vi "1C Camera - find boat given marker locations.vi"(0 "Bow Marker Found":T1, 1 "Bow Marker Location":T3 {"North" format="%#_10f"; "East" format="%#_8f"}, 2 "Bow Marker Heading":T2 format="%05.1f", 3 "Stern Marker Found":T1, 4 "Stern Marker Location":T3 {"North" format="%#_10f"; "East" format="%#_8f"}, 5 "Stern Marker Heading":T2 format="%05.1f") -> (14 "Boat Location":T3 {"North" format="%#_10f"; "East" format="%#_8f"}, 15 "Heading":T2 format="%05.1f", 18 "Boat Found":T1)   [LabVIEW 2011]
doc: "Takes the information from two marker-finders, one for the bow and one for stern of the boat, and uses them to estimate the position of the center of the boat. \nAssumes that the center of the boat is either:\na. halfway in between the markers if both are found\nb. half of a boat length extrapolated in the appropriate direction from the marker that was found, if only one marker was found.\nIf neither marker was found, the Boat Found output will be False and you'll have to look elsewhere for your boat location information, sorry."
uses:
  2-Think/2 Typedefs/UTM Location.ctl
  2-Think/2 Typedefs/heading.ctl
  2-Think/2 Typedefs/indicator LED.ctl
  2-Think/2 Typedefs/Velocity.ctl
panel:
  in  "Distance Bow to Stern (m)":dbl=1.0
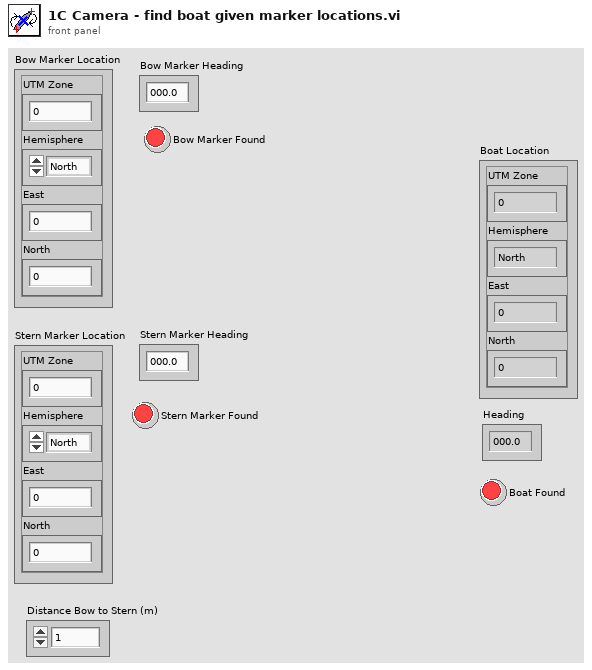
[diagram p1: front panel]
types:
  T1 = typedef "indicator LED.ctl" = bool
  T2 = typedef "heading.ctl" = dbl
  T3 = typedef "UTM Location.ctl" = cluster{"UTM Zone":dbl, "Hemisphere":enum16{"North", "South"}, "East":dbl, "North":dbl}
  T4 = typedef "Velocity.ctl" = cluster{"East":dbl, "North":dbl}
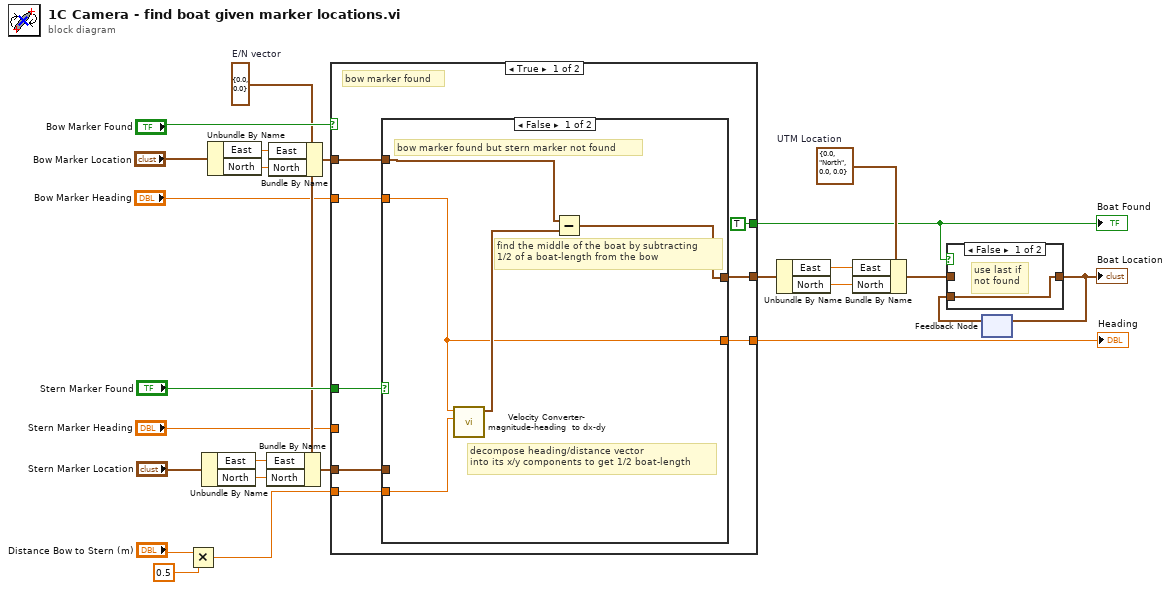
[diagram p0: block diagram]
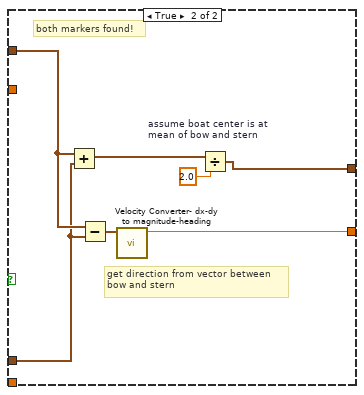
[diagram p3: hidden frame]
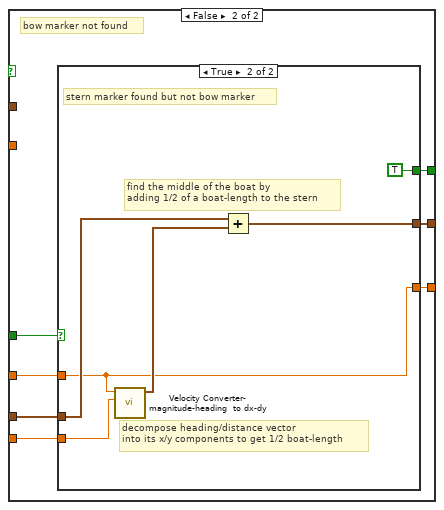
[diagram p4: hidden frame]
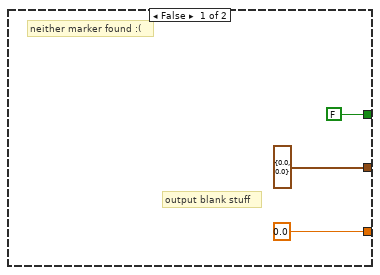
[diagram p5: hidden frame]
diagram:
  w10 = T3 {"UTM Zone"=0.0, "Hemisphere"=enum."North", "East"=0.0, "North"=0.0}  # UTM Location
  w14 = T4 {"East"=0.0, "North"=0.0}  # E/N vector
  n1 = Multiply(x="Distance Bow to Stern (m)", y=0.5) -> (x*y=w7:dbl)
  n2 = Unbundle By Name("Stern Marker Location") -> ("East"=w17:dbl, "North"=w16:dbl)
  n3 = Unbundle By Name("Bow Marker Location") -> ("East"=w19:dbl, "North"=w18:dbl)
  n4 = Bundle By Name(cluster=w14, "East"=w17, "North"=w16) -> (w15:T4)
  n5 = Bundle By Name(cluster=w14, "East"=w19, "North"=w18) -> (w20:T4)
  n6 = case shown="True" "Bow Marker Found" {
    tunnel: "Stern Marker Found" -> [w33 w52]
    tunnel: [TRUE w51] -> w3
    tunnel: [w29 w50] -> w23
    tunnel: w20 -> [w32 _]
    tunnel: w15 -> [w31 w46]
    tunnel: [w28 w49] -> w12
    tunnel: w7 -> [w27 w47]
    tunnel: "Bow Marker Heading" -> [w26 _]
    tunnel: "Stern Marker Heading" -> [_ w48]
    frame True {
      # "bow marker found"
      n7 = case shown="False" w33 {
        tunnel: w32 -> [w37 w43]
        tunnel: w31 -> [_ w42]
        tunnel: [w34 w44] -> w29
        tunnel: [w35 w39] -> w28
        tunnel: w27 -> [w38 _]
        tunnel: w26 -> [w34 _]
        frame False {
          # "decompose heading/distance vector \ninto its x/y components to get 1/2 boat-length"
          # "find the middle of the boat by subtracting \n1/2 of a boat-length from the bow"
          # "bow marker found but stern marker not found"
          n8 = call "Velocity Converter- magnitude-heading  to dx-dy.vi"("Magnitude"=w38, "Heading"=w34) -> ("Vector Out"=w36:T4)  [unwired: 9 in]
          n9 = Subtract(x=w37, y=w36) -> (x-y=w35:T4)
        }
        frame True {
          # "get direction from vector between\nbow and stern"
          # "both markers found!"
          n10 = Add(x=w43, y=w42) -> (x+y=w41:T4)
          n11 = Subtract(x=w43, y=w42) -> (x-y=w45:T4)
          n12 = call "Velocity Converter- dx-dy to magnitude-heading.vi"("Vector In"=w45) -> ("Heading Out"=w44:T2)  [unwired: 9 in, 1 out]
          n13 = Divide "assume boat center is at\nmean of bow and stern"(x=w41, y=2.0) -> (x/y=w39:T4)
        }
      }
    }
    frame False {
      # "bow marker not found"
      n14 = case shown="True" w52 {
        tunnel: [FALSE TRUE] -> w51
        tunnel: [T2 0.0 ("Heading") w56] -> w50
        tunnel: [T4 {"East"=0.0, "North"=0.0} ("E/N vector") w57] -> w49
        tunnel: w48 -> [_ w56]
        tunnel: w47 -> [_ w60]
        tunnel: w46 -> [_ w58]
        frame False {
          # "output blank stuff"
          # "neither marker found :("
        }
        frame True {
          # "find the middle of the boat by\nadding 1/2 of a boat-length to the stern"
          # "decompose heading/distance vector \ninto its x/y components to get 1/2 boat-length"
          # "stern marker found but not bow marker"
          n15 = call "Velocity Converter- magnitude-heading  to dx-dy.vi"("Magnitude"=w60, "Heading"=w56) -> ("Vector Out"=w59:T4)  [unwired: 9 in]
          n16 = Add(x=w58, y=w59) -> (x+y=w57:T4)
        }
      }
    }
  }
  "Heading" <- w23
  "Boat Found" <- w3
  n17 = Unbundle By Name(w12) -> ("East"=w13:dbl, "North"=w11:dbl)
  n18 = Bundle By Name(cluster=w10, "East"=w13, "North"=w11) -> (w4:T3)
  n19 = feedback #1() -> (w1:T3)  [unwired: 1 in]
  n20 = case shown="False" w3 {
    tunnel: [w62 w63] -> w2
    tunnel: w4 -> [_ w63]
    tunnel: w1 -> [w62 _]
    frame False {
      # "use last if \nnot found"
    }
    frame True {
    }
  }
  "Boat Location" <- w2
  n21 = feedback-in #1(w2) -> ()
